vi "SwerveDrive.vi"(0 "x":dbl, 1 "y":dbl, 2 "z":dbl, 3 "z2":dbl, 4 "Yaw":dbl, 5 "Autonomous?":bool, 6 "Robot Centric?":bool=TRUE, 9 "Slow":bool) -> ()   [LabVIEW 2019]
uses:
  <vilib>/Rock Robotics/WPI/ThirdParty/Phoenix-LabVIEW/Motor Controller/Controls/CTRE_Phoenix_MotorControl_ControlMode.ctl
  <vilib>/Rock Robotics/Network Tables/NT Write Numeric Array.vi
  <vilib>/Rock Robotics/WPI/ThirdParty/Phoenix-LabVIEW/Motor Controller/Get/CTRE_Phoenix_MotorController_GetSupplyAndStatorCurrent_Enhanced.vi
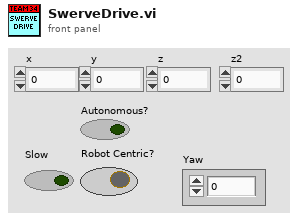
[diagram p1: front panel]
types:
  T1 = typedef "CTRE_Phoenix_MotorControl_ControlMode.ctl" = u16
  T2 = typedef "WPI_MotorControlDeviceRef.ctl" = cluster{"DeviceStatus":errorcluster, "Type":T3, "PWM":cluster{"PWM Channel":T4, "DeadBand":T5}, "CAN":cluster{"Device Number":u8, "SetOutput VI Ref":variant, "GetOutput VI Ref":variant, "Enable VI Ref":variant, "Disable VI Ref":variant, "Data":variant}, "Invert":bool, "DIO PWM":cluster{"PWM \"Enable\" Channel":T4, "DIOChannel":T6, "PWM Rate":dbl}}
  T3 = typedef "WPI_MotorControlType.ctl" = enum16{"PWM", "CAN", "DIO PWM"}
  T4 = typedef "FPGA_DIOPWMChannel.ctl" = enum8{"PWM 0", "PWM 1", "PWM 2", "PWM 3", "PWM 4", "PWM 5", "PWM 6", "PWM 7", "PWM 8", "PWM 9", "PWM MXP 0", "PWM MXP 1", "PWM MXP 2", "PWM MXP 3", "PWM MXP 4", "PWM MXP 5", "PWM MXP 6", "PWM MXP 7", "PWM MXP 8", "PWM MXP 9", "Invalid"}
  T5 = typedef "WPI_PWMDeadband.ctl" = cluster{"Name":string, "maxPositivePwm":i32, "minPositivePwm":i32, "centerPwm":i32, "maxNegativePwm":i32, "minNegativePwm":i32, "angularRange":u16}
  T6 = typedef "FPGA_DIOChannel.ctl" = enum8{"DIO 0", "DIO 1", "DIO 2", "DIO 3", "DIO 4", "DIO 5", "DIO 6", "DIO 7", "DIO 8", "DIO 9", "DIO MXP 0", "DIO MXP 1", "DIO MXP 2", "DIO MXP 3", "DIO MXP 4", "DIO MXP 5", "DIO MXP 6", "DIO MXP 7", "DIO MXP 8", "DIO MXP 9", "DIO MXP 10", "DIO MXP 11", "DIO MXP 12", "DIO MXP 13", "DIO MXP 14", "DIO MXP 15", "SPI Port CS1", "SPI Port CS2", "SPI Port CS3", "SPI Port MISO", "SPI Port MOSI", "Invalid"}
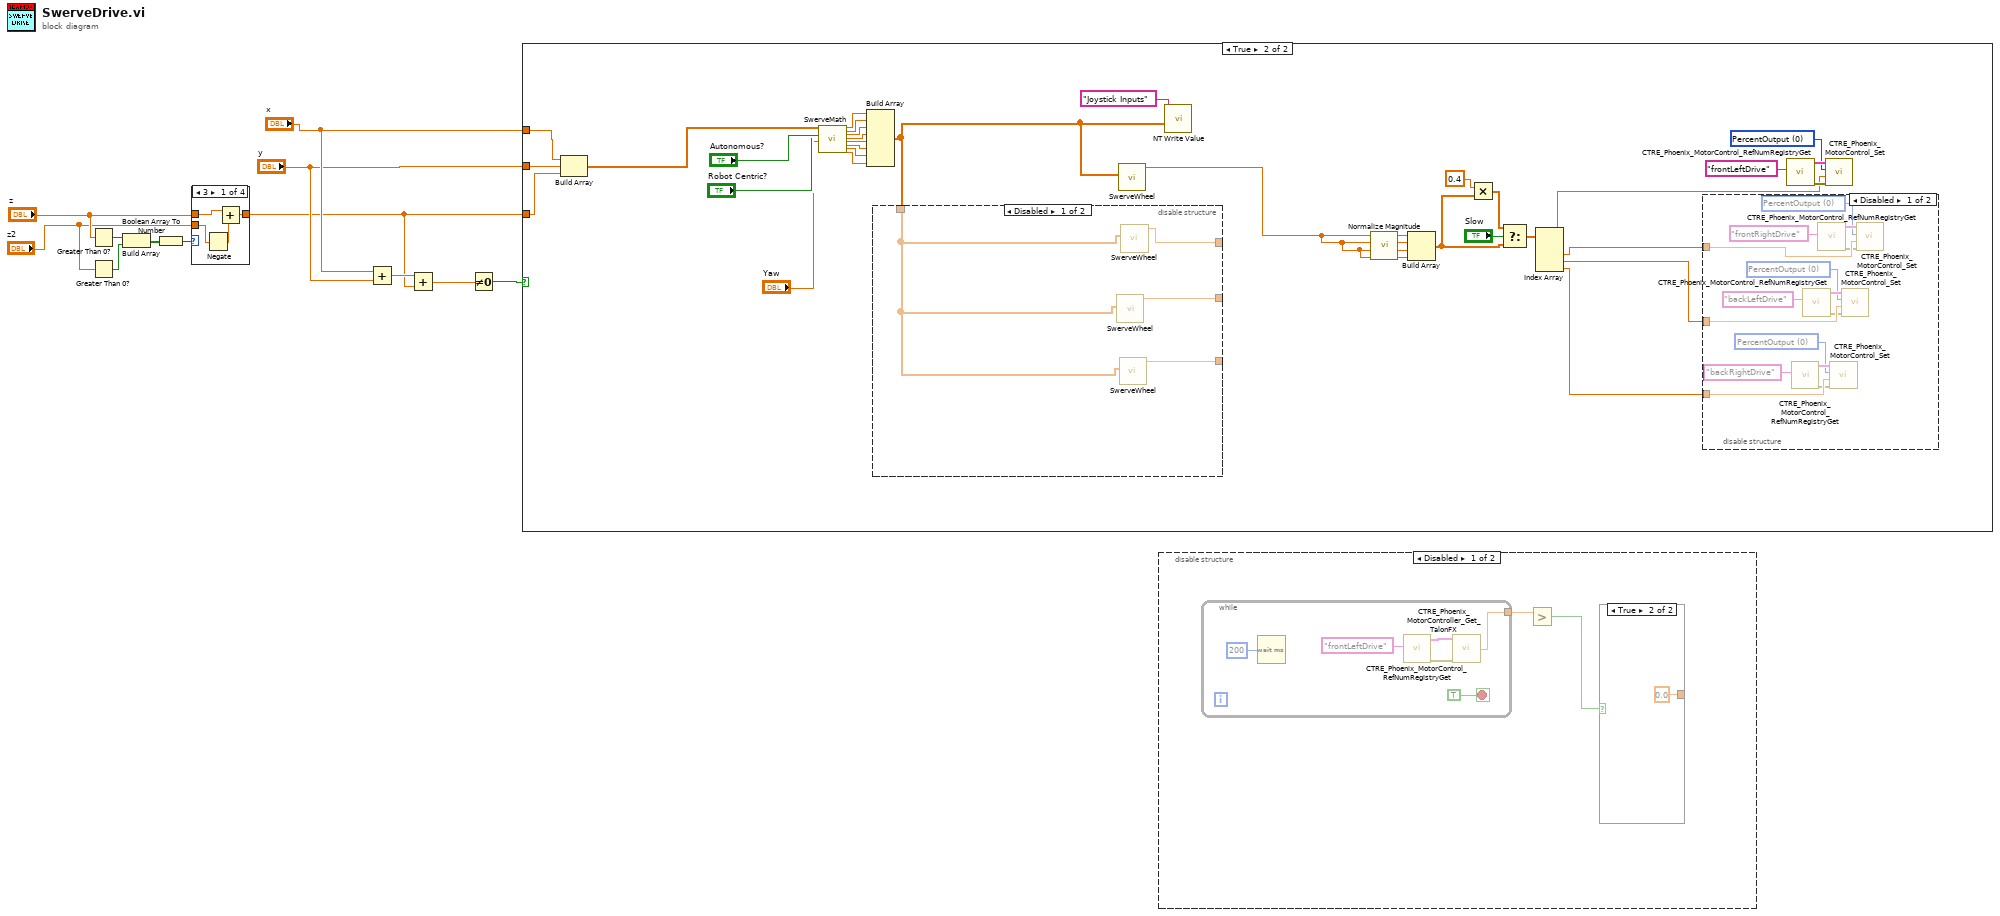
[diagram p0: block diagram]
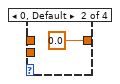
[diagram p2: hidden frame]
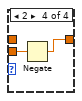
[diagram p4: hidden frame]
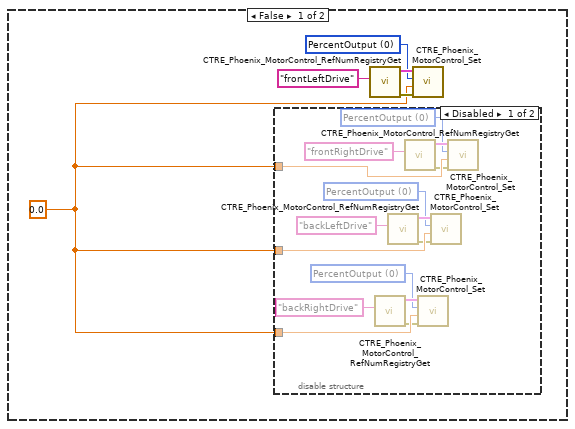
[diagram p5: hidden frame]
diagram:
  n1 = Greater Than 0?(x="z") -> (x > 0?=w11:bool)
  n2 = Greater Than 0?(x="z2") -> (x > 0?=w10:bool)
  n3 = Build Array(w11, w10) -> (w9:bool[])
  n4 = Boolean Array To Number(Boolean array=w9) -> (number=w8:u32)
  n5 = case shown="3" w8 {
    tunnel: [w14 0.0 w18 w19] -> w1
    tunnel: "z" -> [w16 _ w18 _]
    tunnel: "z2" -> [w15 _ _ w20]
    frame 3 {
      n6 = Negate(x=w15) -> (-x=w13:dbl)
      n7 = Add(x=w16, y=w13) -> (x+y=w14:dbl)
    }
    frame 0, Default {
    }
    frame 1 {
    }
    frame 2 {
      n8 = Negate(x=w20) -> (-x=w19:dbl)
    }
  }
  n9 = Add(x="x", y="y") -> (x+y=w5:dbl)
  n10 = Add(x=w5, y=w1) -> (x+y=w4:dbl)
  n11 = Not Equal To 0?(x=w4) -> (x != 0?=w12:bool)
  n12 = case shown="True" w12 {
    tunnel: "x" -> [_ w48]
    tunnel: "y" -> [_ w47]
    tunnel: w1 -> [_ w43]
    frame False {
      w21 = 0.0
      w22 = T1 0 items=["PercentOutput"=0, "Position"=1, "Velocity"=2, "Current"=3, "Follower"=5, "MotionProfile"=6, "MotionMagic"=7, "MotionProfileArc"=10, "Disabled"=15] ("Control Mode")
      n13 = disable-structure shown="Disabled" {
        disable-tunnel: w21 -> [w40 _]
        disable-tunnel: w21 -> [w39 _]
        disable-tunnel: w21 -> [w38 _]
        frame Disabled {
          w26 = T1 0 items=["PercentOutput"=0, "Position"=1, "Velocity"=2, "Current"=3, "Follower"=5, "MotionProfile"=6, "MotionMagic"=7, "MotionProfileArc"=10, "Disabled"=15] ("Control Mode")
          w27 = T1 0 items=["PercentOutput"=0, "Position"=1, "Velocity"=2, "Current"=3, "Follower"=5, "MotionProfile"=6, "MotionMagic"=7, "MotionProfileArc"=10, "Disabled"=15] ("Control Mode")
          w28 = T1 0 items=["PercentOutput"=0, "Position"=1, "Velocity"=2, "Current"=3, "Follower"=5, "MotionProfile"=6, "MotionMagic"=7, "MotionProfileArc"=10, "Disabled"=15] ("Control Mode")
          n14 = call <vilib>:"CTRE_Phoenix_MotorControl_RefNumRegistryGet.vi"("refnum name"="backRightDrive") -> ("error out"=w36:errorcluster, "PhoenixMotorControlDevRef"=w37:T2)  [unwired: 9 in]
          n15 = call <vilib>:"CTRE_Phoenix_MotorControl_RefNumRegistryGet.vi"("refnum name"="backLeftDrive") -> ("error out"=w34:errorcluster, "PhoenixMotorControlDevRef"=w35:T2)  [unwired: 9 in]
          n16 = call <vilib>:"CTRE_Phoenix_MotorControl_RefNumRegistryGet.vi"("refnum name"="frontRightDrive") -> ("error out"=w32:errorcluster, "PhoenixMotorControlDevRef"=w33:T2)  [unwired: 9 in]
          n17 = call <vilib>:"CTRE_Phoenix_MotorControl_Set.vi"("error in (no error)"=w36, "Output"=w38, "Control Mode"=w26, "PhoenixMotorControlDevRef"=w37) -> ()  [unwired: 6 in, 2 out]
          n18 = call <vilib>:"CTRE_Phoenix_MotorControl_Set.vi"("error in (no error)"=w34, "Output"=w39, "Control Mode"=w27, "PhoenixMotorControlDevRef"=w35) -> ()  [unwired: 6 in, 2 out]
          n19 = call <vilib>:"CTRE_Phoenix_MotorControl_Set.vi"("error in (no error)"=w32, "Output"=w40, "Control Mode"=w28, "PhoenixMotorControlDevRef"=w33) -> ()  [unwired: 6 in, 2 out]
        }
        frame Enabled {
        }
      }
      n20 = call <vilib>:"CTRE_Phoenix_MotorControl_RefNumRegistryGet.vi"("refnum name"="frontLeftDrive") -> ("error out"=w24:errorcluster, "PhoenixMotorControlDevRef"=w25:T2)  [unwired: 9 in]
      n21 = call <vilib>:"CTRE_Phoenix_MotorControl_Set.vi"("error in (no error)"=w24, "Output"=w21, "Control Mode"=w22, "PhoenixMotorControlDevRef"=w25) -> ()  [unwired: 6 in, 2 out]
    }
    frame True {
      w55 = T1 0 items=["PercentOutput"=0, "Position"=1, "Velocity"=2, "Current"=3, "Follower"=5, "MotionProfile"=6, "MotionMagic"=7, "MotionProfileArc"=10, "Disabled"=15] ("Control Mode")
      n22 = Build Array(w48, w47, w43) -> (w52:dbl[])
      n23 = call "SwerveMath.vi"("Inputs"=w52, "Autonomous?"="Autonomous?", "Robot Centric?"="Robot Centric?", "Yaw"="Yaw") -> ("wheelSpeed1"=w75:dbl, "wheelSpeed2"=w74:dbl, "wheelSpeed3"=w73:dbl, "wheelSpeed4"=w72:dbl, "wheelAngle1"=w71:dbl, "wheelAngle2"=w70:dbl, "wheelAngle3"=w69:dbl, "wheelAngle4"=w68:dbl)  [unwired: 16 in]
      n24 = Build Array(w75, w74, w73, w72, w71, w70, w69, w68) -> (w50:dbl[])
      n25 = disable-structure shown="Disabled" {
        disable-tunnel: [w94 _] -> _
        disable-tunnel: [w93 _] -> _
        disable-tunnel: [w92 _] -> _
        disable-tunnel: w50 -> [w91 _]
        frame Disabled {
          n26 = call "SwerveWheel.vi"("Inputs"=w91) -> ("Speed"=w93:dbl)  [unwired: 9 in, 1 out]
          n27 = call "SwerveWheel.vi"("Inputs"=w91) -> ("Speed"=w92:dbl)  [unwired: 9 in, 1 out]
          n28 = call "SwerveWheel.vi"("Inputs"=w91) -> ("Speed"=w94:dbl)  [unwired: 9 in, 1 out]
        }
        frame Enabled {
        }
      }
      n29 = call "SwerveWheel.vi"("Inputs"=w50) -> ("Speed"=w41:dbl)  [unwired: 9 in, 1 out]
      n30 = call-poly <vilib>:"NT Write Value.vi"("Numeric Array"=w50, "Name"="Joystick Inputs") -> ()  [unwired: 9 in, 1 out]
      n31 = call "Normalize Magnitude.vi"("D"=w41, "C"=w41, "B"=w41, "A"=w41) -> ("D'"=w59:dbl, "C'"=w60:dbl, "B'"=w61:dbl, "A'"=w62:dbl)  [unwired: 4 in]
      n32 = Build Array(w62, w61, w60, w59) -> (w65:dbl[])
      n33 = Multiply(x=0.4, y=w65) -> (x*y=w63:dbl[])
      n34 = Select(t=w63, s="Slow", f=w65) -> (s? t:f=w67:dbl[])
      n35 = Index Array(array=w67) -> (element #1=w42:dbl, element #2=w46:dbl, element #3=w45:dbl, element #4=w44:dbl)  [unwired: 4 in]
      n36 = disable-structure shown="Disabled" {
        disable-tunnel: w46 -> [w90 _]
        disable-tunnel: w45 -> [w89 _]
        disable-tunnel: w44 -> [w88 _]
        frame Disabled {
          w76 = T1 0 items=["PercentOutput"=0, "Position"=1, "Velocity"=2, "Current"=3, "Follower"=5, "MotionProfile"=6, "MotionMagic"=7, "MotionProfileArc"=10, "Disabled"=15] ("Control Mode")
          w77 = T1 0 items=["PercentOutput"=0, "Position"=1, "Velocity"=2, "Current"=3, "Follower"=5, "MotionProfile"=6, "MotionMagic"=7, "MotionProfileArc"=10, "Disabled"=15] ("Control Mode")
          w78 = T1 0 items=["PercentOutput"=0, "Position"=1, "Velocity"=2, "Current"=3, "Follower"=5, "MotionProfile"=6, "MotionMagic"=7, "MotionProfileArc"=10, "Disabled"=15] ("Control Mode")
          n37 = call <vilib>:"CTRE_Phoenix_MotorControl_RefNumRegistryGet.vi"("refnum name"="backRightDrive") -> ("error out"=w86:errorcluster, "PhoenixMotorControlDevRef"=w87:T2)  [unwired: 9 in]
          n38 = call <vilib>:"CTRE_Phoenix_MotorControl_RefNumRegistryGet.vi"("refnum name"="backLeftDrive") -> ("error out"=w84:errorcluster, "PhoenixMotorControlDevRef"=w85:T2)  [unwired: 9 in]
          n39 = call <vilib>:"CTRE_Phoenix_MotorControl_RefNumRegistryGet.vi"("refnum name"="frontRightDrive") -> ("error out"=w82:errorcluster, "PhoenixMotorControlDevRef"=w83:T2)  [unwired: 9 in]
          n40 = call <vilib>:"CTRE_Phoenix_MotorControl_Set.vi"("error in (no error)"=w86, "Output"=w88, "Control Mode"=w76, "PhoenixMotorControlDevRef"=w87) -> ()  [unwired: 6 in, 2 out]
          n41 = call <vilib>:"CTRE_Phoenix_MotorControl_Set.vi"("error in (no error)"=w84, "Output"=w89, "Control Mode"=w77, "PhoenixMotorControlDevRef"=w85) -> ()  [unwired: 6 in, 2 out]
          n42 = call <vilib>:"CTRE_Phoenix_MotorControl_Set.vi"("error in (no error)"=w82, "Output"=w90, "Control Mode"=w78, "PhoenixMotorControlDevRef"=w83) -> ()  [unwired: 6 in, 2 out]
        }
        frame Enabled {
        }
      }
      n43 = call <vilib>:"CTRE_Phoenix_MotorControl_RefNumRegistryGet.vi"("refnum name"="frontLeftDrive") -> ("error out"=w57:errorcluster, "PhoenixMotorControlDevRef"=w58:T2)  [unwired: 9 in]
      n44 = call <vilib>:"CTRE_Phoenix_MotorControl_Set.vi"("error in (no error)"=w57, "Output"=w42, "Control Mode"=w55, "PhoenixMotorControlDevRef"=w58) -> ()  [unwired: 6 in, 2 out]
    }
  }
  n45 = disable-structure shown="Disabled" {
    frame Disabled {
      n46 = while {
        tunnel: [w97] -> w95
        stop <- TRUE stop-if-true
        n47 = Wait (ms)(milliseconds to wait=u32 200) -> ()  [unwired: 1 out]
        n48 = call <vilib>:"CTRE_Phoenix_MotorControl_RefNumRegistryGet.vi"("refnum name"="frontLeftDrive") -> ("error out"=w99:errorcluster, "PhoenixMotorControlDevRef"=w100:T2)  [unwired: 9 in]
        n49 = call-poly <vilib>:"CTRE_Phoenix_MotorController_Get_TalonFX.vi"("PhoenixMotorControlDevRef"=w100, "error in"=w99) -> ("Stator Current"=w97:dbl)  [unwired: 10 in, 3 out]
      }
      n50 = Greater?(x=w95) -> (0:w96:bool)  [unwired: 1 in]
      n51 = case shown="True" w96 {
        tunnel: [_ 0.0 ("D'")] -> _
        frame False {
        }
        frame True {
        }
      }
    }
    frame Enabled {
    }
  }
